vi "Multiple Straight Line Moves.vi"() -> ()   [LabVIEW 2014]
doc: "This example shows a single axis straight-line move using the NI SoftMotion Line function block.\n\nNote: You must have the LabVIEW NI SoftMotion Module installed to run this example."
uses:
  <vilib>/Motion/Express/_s/nimc.fb.straightLineMove.startStraightLineMove.axis.modeRelative.0.vi
  <vilib>/Motion/Express/_s/nimc.fb.stopMove.stop.axis.modeDecelerate.vi
  <vilib>/Motion/Express/_s/nimc.fb.read.readExecutionData.axis.vi
  <vilib>/Motion/BlockNode/FB.NIMotion.xnode
panel:
  out "Acceleration (decimicrons/s2)":dbl
  out "Velocity (decimicrons/s)":dbl
  out "Position at Peak (decimicrons)":dbl
  in  "Target Peak Displacement (mm)":dbl=2.0
  in  "Target Pulse Duration (ms)":dbl=1000.0
  out "Single Plot (Array of X,Y Pairs)":cluster{u32[], dbl[]}(graph)
  out "Example Done":bool=TRUE
  out "error out":errorcluster={"status"=FALSE, "code"=77003, "source"="Invoke Node in nimc.fb.straightLineMove.startStraightLineMove.axis.modeAbsolute.0.vi:5060005->Multiple Straight Line Moves.vi"}
  in  "Resource":refnum<k21>="Axis 1"
  # "Computed Inputs"
  # "Target Parameters"
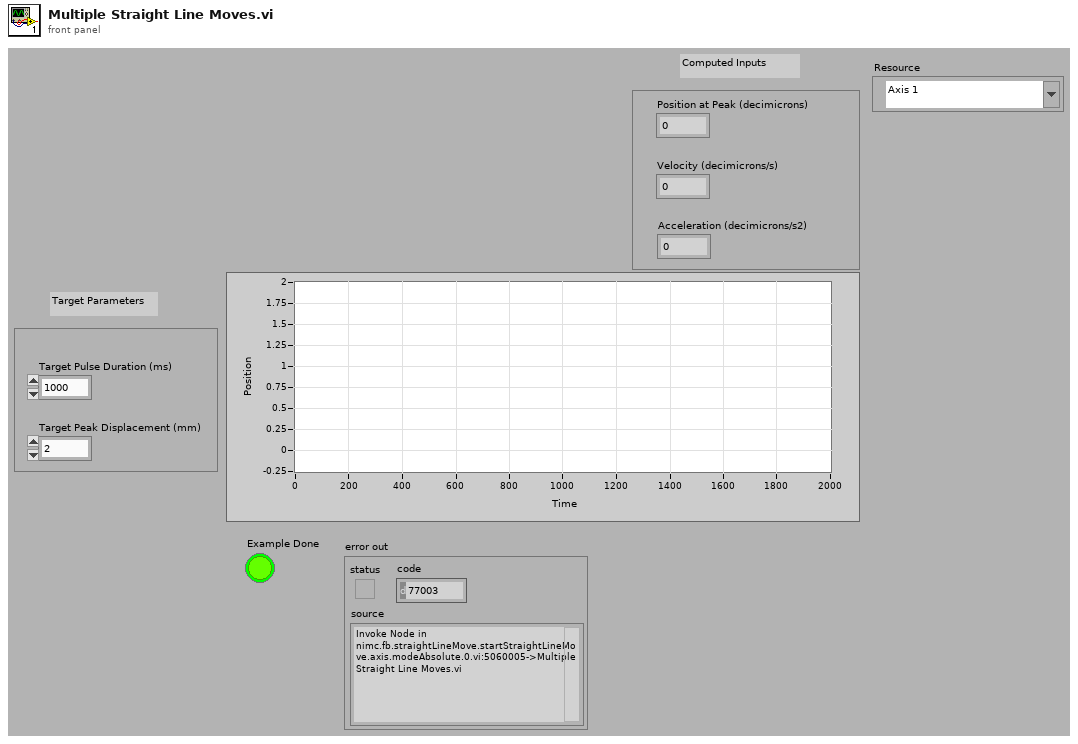
[diagram p1: front panel]
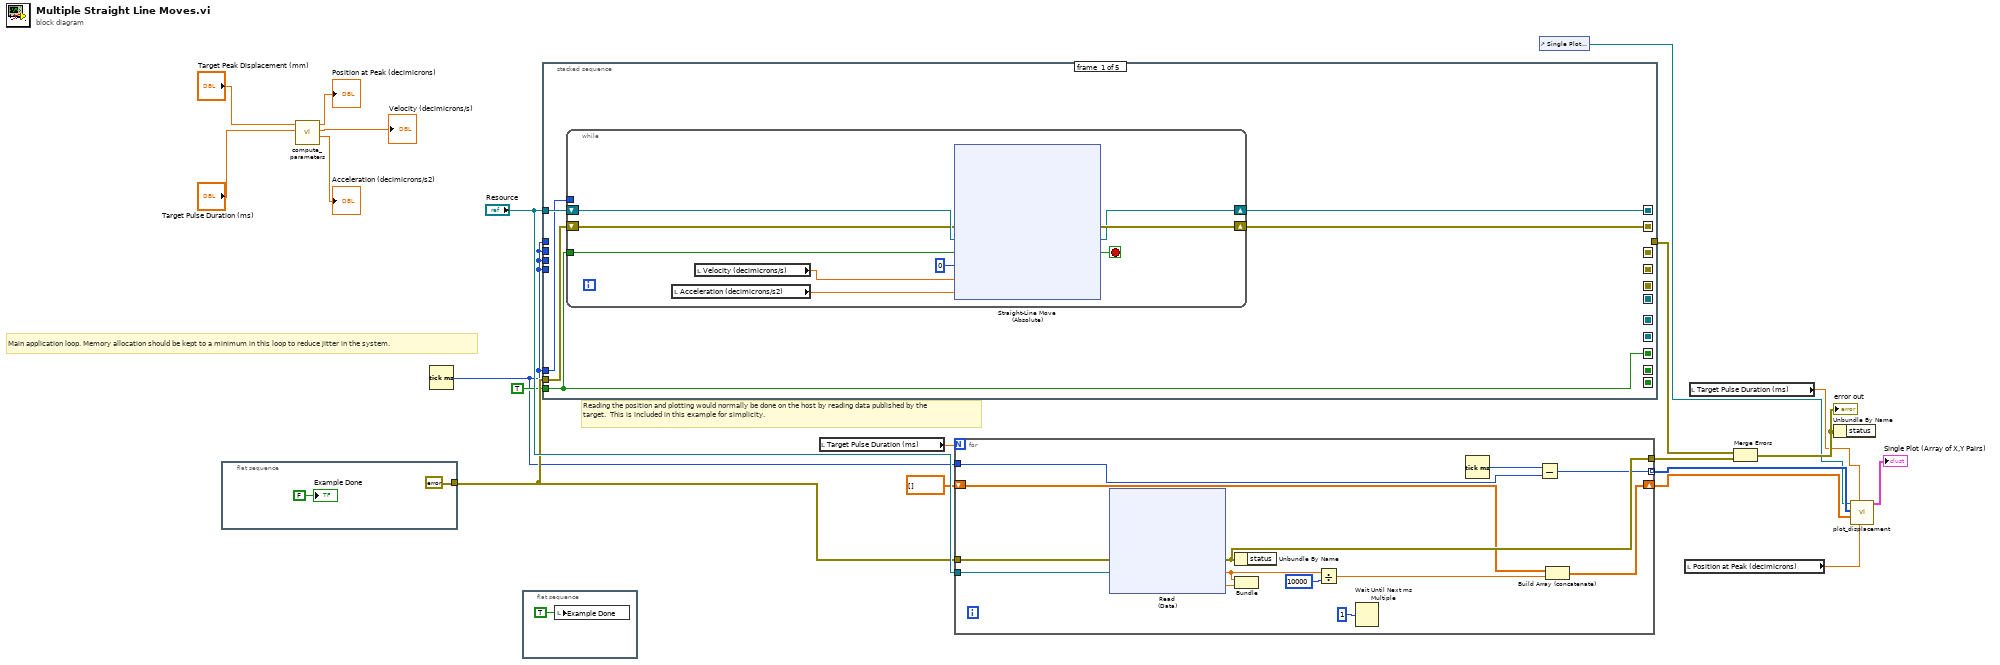
[diagram p0: block diagram]
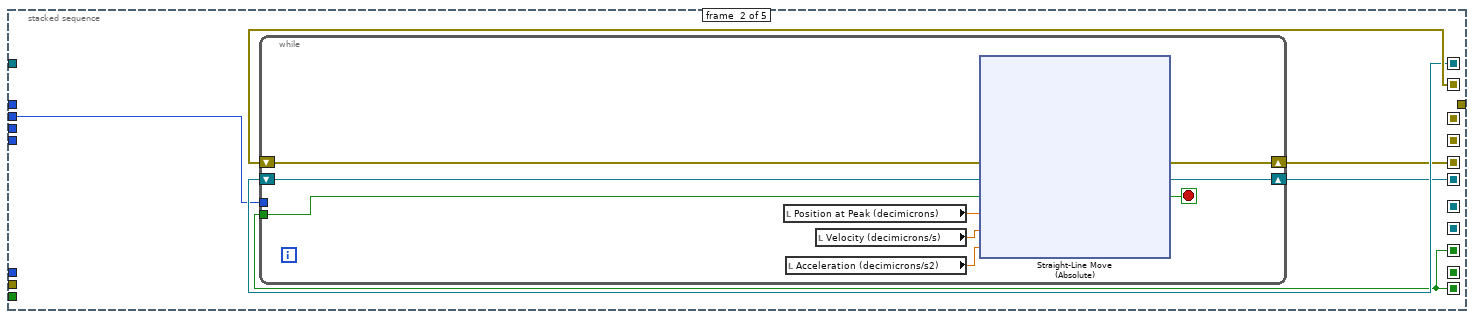
[diagram p2: hidden frame]
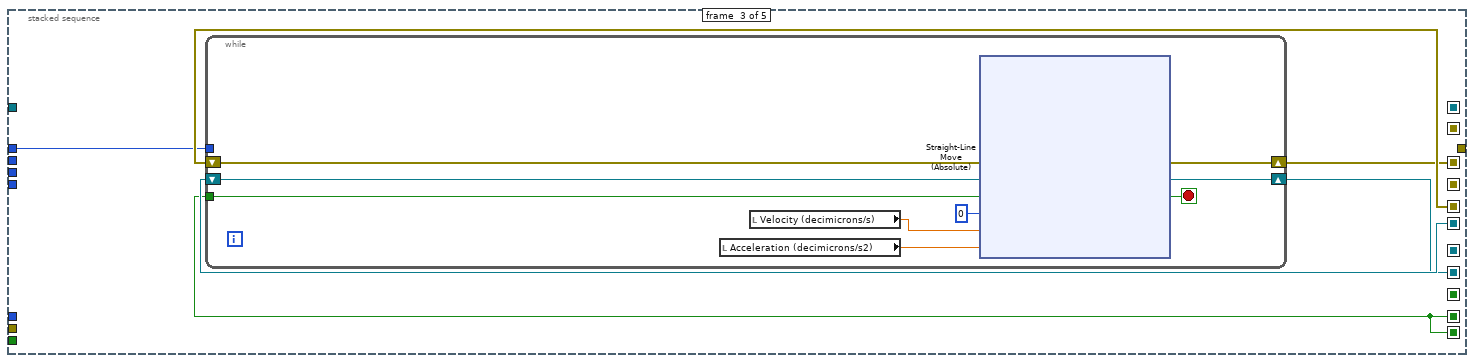
[diagram p3: hidden frame]
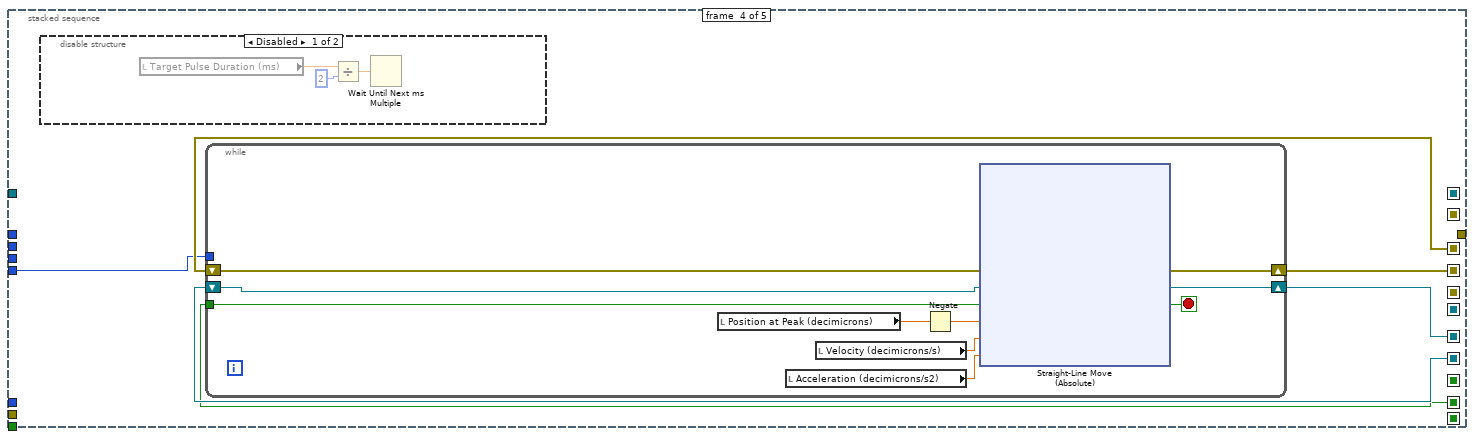
[diagram p4: hidden frame]
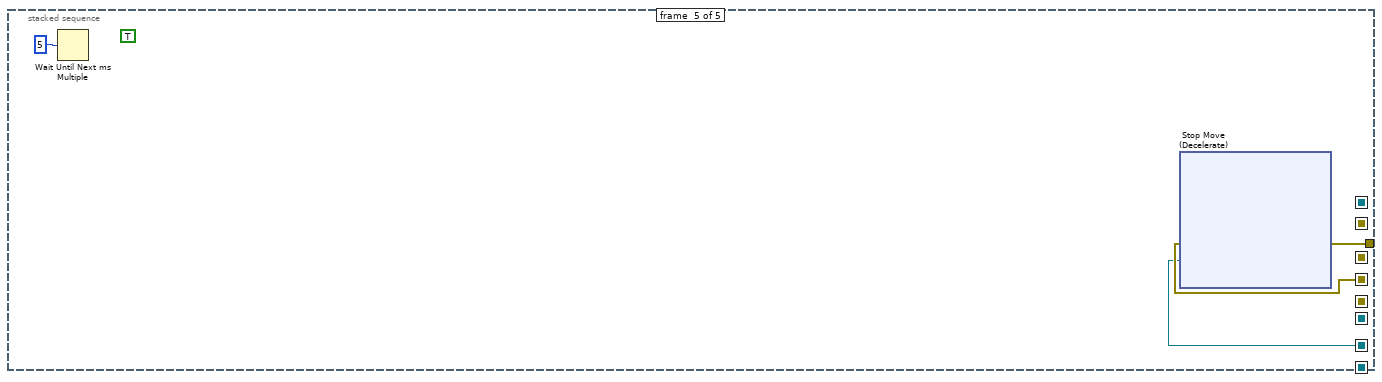
[diagram p6: hidden frame]
diagram:
  # "Reading the position and plotting would normally be done on the host by reading data published by the target.  This is included in this example for simplicity."
  # "Main application loop. Memory allocation should be kept to a minimum in this loop to reduce jitter in the system."
  n1 = flat-sequence {
    tunnel: [errorcluster {"status"=FALSE, "code"=0, "source"=""} ("Error")] -> w19
    frame #0 {
      "Example Done" <- FALSE ("Example Done")
    }
  }
  n2 = call "compute_parameters.vi"("Target Pulse Duration (ms)"="Target Pulse Duration (ms)", "Target Peak Displacement (mm)"="Target Peak Displacement (mm)") -> ("Acceleration (decimicrons/s2)"=→"Acceleration (decimicrons/s2)":dbl, "Velocity (decimicrons/s)"=→"Velocity (decimicrons/s)":dbl, "Position at Peak (decimicrons)"=→"Position at Peak (decimicrons)":dbl)  [unwired: 7 in]
  n3 = Tick Count (ms)() -> (millisecond timer value=w14:u32)
  n4 = flat-sequence {
    frame #0 {
      n5 = local write "Example Done"(TRUE ("Example Done")) -> ()
    }
  }
  n6 = stacked-sequence {
    seq-local: [w27 _ _ _ _] -> [_ w61 _ _ _]
    seq-local: [w26 _ _ _ _] -> [_ w60 _ _ _]
    seq-local: [w25 _ _ _ _] -> [_ w57 _ _ _]
    seq-local: [_ w59 _ _ _] -> [_ _ w93 _ _]
    seq-local: [_ w58 _ _ _] -> [_ _ w91 _ _]
    seq-local: [_ w57 _ _ _] -> [_ _ w89 _ _]
    seq-local: [_ _ w92 _ _] -> [_ _ _ w125 _]
    seq-local: [_ _ w90 _ _] -> [_ _ _ w123 _]
    seq-local: [_ _ w89 _ _] -> [_ _ _ w121 _]
    seq-local: [_ _ _ w124 _] -> [_ _ _ _ w159]
    seq-local: [_ _ _ w122 _] -> [_ _ _ _ w157]
    tunnel: "Resource" -> [w29 _ _ _ _]
    tunnel: w19 -> [w28 _ _ _ _]
    tunnel: TRUE ("approach forward") -> [w25 _ _ _ _]
    tunnel: w14 -> [w24 _ _ _ _]
    tunnel: w14 -> [_ w56 _ _ _]
    tunnel: w14 -> [_ _ w88 _ _]
    tunnel: w14 -> [_ _ _ w120 _]
    tunnel: [_ _ _ _ w158] -> w16
    tunnel: w14 -> [_ _ _ _ _]
    frame #0 {
      n7 = while {
        tunnel: w25 -> [w34]
        tunnel: w24 -> [_]
        shift-right: [w35] -> w26
        shift-left: w29 -> [w38]
        shift-right: [w36] -> w27
        shift-left: w28 -> [w37]
        stop <- w33 stop-if-true
        n8 = local read "Acceleration (decimicrons/s2)"() -> (w30:dbl)
        n9 = local read "Velocity (decimicrons/s)"() -> (w31:dbl)
        n10 = xnode "Straight-Line Move\n(Absolute)"("error in"=w37, "resource"=w38, "execute"=w34, "position"=0, "velocity"=w31, "acceleration"=w30) -> ("error out"=w36:errorcluster, "resource out"=w35:refnum<k21>, "done"=w33:bool)
      }
    }
    frame #1 {
      n11 = while {
        tunnel: w57 -> [w66]
        tunnel: w56 -> [_]
        shift-right: [w68] -> w59
        shift-left: w61 -> [w70]
        shift-right: [w67] -> w58
        shift-left: w60 -> [w69]
        stop <- w62 stop-if-true
        n12 = local read "Position at Peak (decimicrons)"() -> (w65:dbl)
        n13 = local read "Acceleration (decimicrons/s2)"() -> (w63:dbl)
        n14 = local read "Velocity (decimicrons/s)"() -> (w64:dbl)
        n15 = xnode "Straight-Line Move\n(Absolute)"("error in"=w70, "resource"=w69, "execute"=w66, "position"=w65, "velocity"=w64, "acceleration"=w63) -> ("error out"=w68:errorcluster, "resource out"=w67:refnum<k21>, "done"=w62:bool)
      }
    }
    frame #2 {
      n16 = while {
        tunnel: w89 -> [w98]
        tunnel: w88 -> [_]
        shift-right: [w101] -> w92
        shift-left: w93 -> [w102]
        shift-right: [w99] -> w90
        shift-left: w91 -> [w100]
        stop <- w94 stop-if-true
        n17 = local read "Acceleration (decimicrons/s2)"() -> (w96:dbl)
        n18 = local read "Velocity (decimicrons/s)"() -> (w97:dbl)
        n19 = xnode "Straight-Line Move\n(Absolute)"("error in"=w102, "resource"=w100, "execute"=w98, "position"=0, "velocity"=w97, "acceleration"=w96) -> ("error out"=w101:errorcluster, "resource out"=w99:refnum<k21>, "done"=w94:bool)
      }
    }
    frame #3 {
      n20 = disable-structure shown="Disabled" {
        frame Disabled {
          n21 = local read "Target Pulse Duration (ms)"() -> (w126:dbl)
          n22 = Divide(x=w126, y=2) -> (x/y=w127:dbl)
          n23 = Wait Until Next ms Multiple(millisecond multiple=w127) -> ()  [unwired: 1 out]
        }
        frame Enabled {
        }
      }
      n24 = while {
        tunnel: w121 -> [w134]
        tunnel: w120 -> [_]
        shift-right: [w137] -> w124
        shift-left: w125 -> [w138]
        shift-right: [w135] -> w122
        shift-left: w123 -> [w136]
        stop <- w129 stop-if-true
        n25 = local read "Position at Peak (decimicrons)"() -> (w131:dbl)
        n26 = local read "Acceleration (decimicrons/s2)"() -> (w132:dbl)
        n27 = local read "Velocity (decimicrons/s)"() -> (w133:dbl)
        n28 = Negate(x=w131) -> (-x=w130:dbl)
        n29 = xnode "Straight-Line Move\n(Absolute)"("error in"=w138, "resource"=w136, "execute"=w134, "position"=w130, "velocity"=w133, "acceleration"=w132) -> ("error out"=w137:errorcluster, "resource out"=w135:refnum<k21>, "done"=w129:bool)
      }
    }
    frame #4 {
      (unwired) TRUE
      n30 = Wait Until Next ms Multiple(millisecond multiple=u32 5) -> ()  [unwired: 1 out]
      n31 = xnode "Stop Move\n(Decelerate)"("error in"=w159, "resource"=w157) -> ("error out"=w158:errorcluster)  [unwired: 1 in, 1 out]
    }
  }
  n32 = local read "Target Pulse Duration (ms)"() -> (w12:dbl)
  n33 = for {
    N: w12 -> [_]
    tunnel: "Resource" -> [w178]
    tunnel: w19 -> [w179]
    tunnel: [w176] -> w18
    tunnel: w14 -> [w174]
    shift-right: [w170] -> w4
    shift-left: dbl[] [] -> [w171]
    tunnel: [w167] -> w3 mode=indexing
    n34 = xnode "Read\n(Data)"("error in"=w179, "resource"=w178) -> ("error out"=w176:errorcluster, "position"=w172:dbl, "velocity"=w177:dbl)
    n35 = Unbundle By Name(w176) -> ()  [unwired: 1 out]
    n36 = Bundle("position"=w172, "velocity"=w177) -> ()  [unwired: 2 out]
    n37 = Divide(x=w172, y=10000) -> (x/y=w169:dbl)
    n38 = Wait Until Next ms Multiple(millisecond multiple=u32 1) -> ()  [unwired: 1 out]
    n39 = Tick Count (ms)() -> (millisecond timer value=w175:u32)
    n40 = Subtract(x=w175, y=w174) -> (x-y=w167:u32)
    n41 = Build Array (concatenate)(w171, w169) -> (w170:dbl[])
  }
  n42 = control-ref of="Single Plot (Array of X,Y Pairs)"() -> (w1:refnum<vi>)
  n43 = local read "Position at Peak (decimicrons)"() -> (w5:dbl)
  n44 = local read "Target Pulse Duration (ms)"() -> (w2:dbl)
  n45 = Merge Errors(w16, w18) -> (w15:errorcluster)
  "error out" <- w15
  n46 = Unbundle By Name(w15) -> ()  [unwired: 1 out]
  n47 = call "plot_displacement.vi"("Position at Peak (decimicrons)"=w5, "Target Pulse Duration (ms)"=w2, "Array"=w4, "Array 2"=w3, "XYGraph in"=w1) -> ("Cluster"=→"Single Plot (Array of X,Y Pairs)":cluster{u32[], dbl[]})  [unwired: 6 in]
